vi "keyboard.NoteOn.vi"(8 "error in (no error)":errorcluster, 10 "Note":T1, 11 "midi-ui in":refnum<class "midi-ui.lvclass">) -> (0 "error out":errorcluster, 3 "midi-ui out":refnum<class "midi-ui.lvclass">)   [LabVIEW 2020, in "midi-ui.lvclass"]
uses:
  midi-ui.lvclass
  shared/midi note number.ctl
  midi-ui.lvclass/midi-ui.ctl
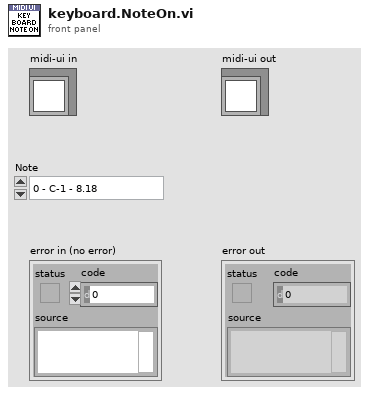
[diagram p1: front panel]
types:
  T1 = typedef "midi note number.ctl" = enum8{"0 - C-1 - 8.18", "1 - C#-1 - 8.66", "2 - D-1 - 9.18", "3 - D#-1 - 9.72", "4 - E-1 - 10.30", "5 - F-1 - 10.91", "6 - F#-1 - 11.56", "7 - G-1 - 12.25", "8 - G#-1 - 12.98", "9 - A-1 - 13.75", "10 - A#-1 - 14.57", "11 - B-1 - 15.43", "12 - C0 - 16.35", "13 - C#0 - 17.32", "14 - D0 - 18.35", "15 - D#0 - 19.45", "16 - E0 - 20.60", "17 - F0 - 21.83", "18 - F#0 - 23.12", "19 - G0 - 24.50", "20 - G#0 - 25.96", "21 - A0 - 27.50", "22 - A#0 - 29.14", "23 - B0 - 30.87", "24 - C1 - 32.70", "25 - C#1 - 34.65", "26 - D1 - 36.71", "27 - D#1 - 38.89", "28 - E1 - 41.20", "29 - F1 - 43.65", "30 - F#1 - 46.25", "31 - G1 - 49.00", "32 - G#1 - 51.91", "33 - A1 - 55.00", "34 - A#1 - 58.27", "35 - B1 - 61.74", "36 - C2 - 65.41", "37 - C#2 - 69.30", "38 - D2 - 73.42", "39 - D#2 - 77.78", "40 - E2 - 82.41", "41 - F2 - 87.31", "42 - F#2 - 92.50", "43 - G2 - 98.00", "44 - G#2 - 103.83", "45 - A2 - 110.00", "46 - A#2 - 116.54", "47 - B2 - 123.47", "48 - C3 - 130.81", "49 - C#3 - 138.59", "50 - D3 - 146.83", "51 - D#3 - 155.56", "52 - E3 - 164.81", "53 - F3 - 174.61", "54 - F#3 - 185.00", "55 - G3 - 196.00", "56 - G#3 - 207.65", "57 - A3 - 220.00", "58 - A#3 - 233.08", "59 - B3 - 246.94", "60 - C4 - 261.63", "61 - C#4 - 277.18", "62 - D4 - 293.66", "63 - D#4 - 311.13", "64 - E4 - 329.63", "65 - F4 - 349.23", "66 - F#4 - 369.99", "67 - G4 - 392.00", "68 - G#4 - 415.30", "69 - A4 - 440.00", "70 - A#4 - 466.16", "71 - B4 - 493.88", "72 - C5 - 523.25", "73 - C#5 - 554.37", "74 - D5 - 587.33", "75 - D#5 - 622.25", "76 - E5 - 659.25", "77 - F5 - 698.46", "78 - F#5 - 739.99", "79 - G5 - 783.99", "80 - G#5 - 830.61", "81 - A5 - 880.00", "82 - A#5 - 932.33", "83 - B5 - 987.77", "84 - C6 - 1046.50", "85 - C#6 - 1108.73", "86 - D6 - 1174.66", "87 - D#6 - 1244.51", "88 - E6 - 1318.51", "89 - F6 - 1396.91", "90 - F#6 - 1479.98", "91 - G6 - 1567.98", "92 - G#6 - 1661.22", "93 - A6 - 1760.00", "94 - A#6 - 1864.66", "95 - B6 - 1975.53", "96 - C7 - 2093.00", "97 - C#7 - 2217.46", "98 - D7 - 2349.32", "99 - D#7 - 2489.02", "100 - E7 - 2637.02", "101 - F7 - 2793.83", "102 - F#7 - 2959.96", "103 - G7 - 3135.96", "104 - G#7 - 3322.44", "105 - A7 - 3520.00", "106 - A#7 - 3729.31", "107 - B7 - 3951.07", "108 - C8 - 4186.01", "109 - C#8 - 4434.92", "110 - D8 - 4698.63", "111 - D#8 - 4978.03", "112 - E8 - 5274.04", "113 - F8 - 5587.65", "114 - F#8 - 5919.91", "115 - G8 - 6271.93", "116 - G#8 - 6644.88", "117 - A8 - 7040.00", "118 - A#8 - 7458.62", "119 - B8 - 7902.13", "120 - C9 - 8372.02", "121 - C#9 - 8869.84", "122 - D9 - 9397.27", "123 - D#9 - 9956.06", "124 - E9 - 10548.08", "125 - F9 - 11175.30", "126 - F#9 - 11839.82", "127 - G9 - 12543.85"}
  T2 = typedef "midi-ui.lvclass/privatedata.ctl" = cluster{"White Key Length":dbl, "White Key Width":dbl, "Black Key Length":dbl, "Key Polygon Corners by Name":map{string, cluster{"x":dbl, "y":dbl}[]}, "Anticlockwise rotations [0-3] (0)":i32, "Polygon Corners by Note Name":map{T1, cluster{"x":dbl, "y":dbl}[]}, "Picture Control":refnum<vi>, "Owning VI":refnum<vi>, "Control Index":i32, "Keyboard Key Note Bounds by Note Name":map{T1, cluster{"max":dbl, "min":dbl}}, "Notes on screen":cluster{"Note":T1, "End Time":u32, "Start Time":u32}[], "Polygon Pictures by Note Name":map{T1, cluster{"Note On":picture, "Note Off":picture}}, "keyboard":picture[], "Keyboard Note Picture Index by Name":map{T1, i32}, "music":picture[], "Zoom Factor":sgl, "keyboard - all off":picture[]}
  T3 = map{T1, cluster{"Note On":picture, "Note Off":picture}}
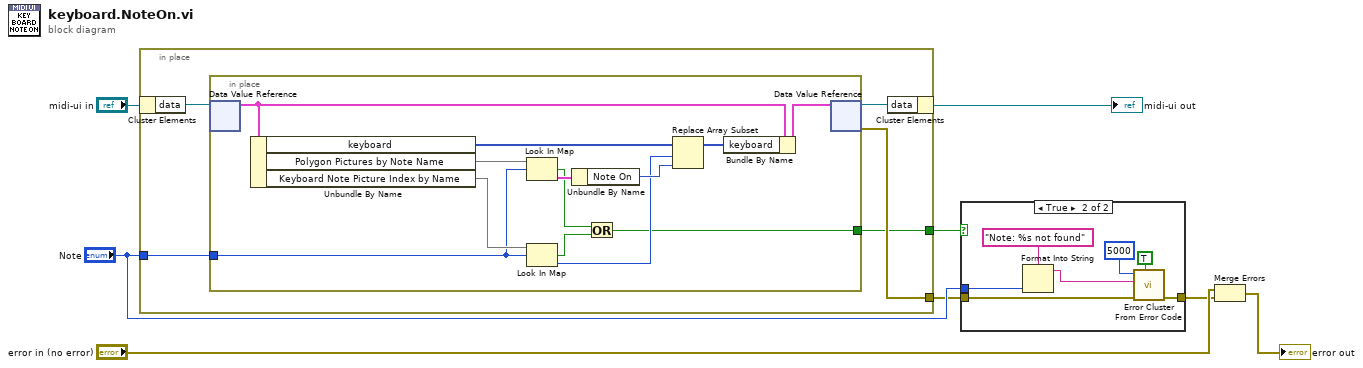
[diagram p0: block diagram]
diagram:
  n1 = in-place {
    in-place-border: "Note" -> [w13]
    in-place-border: [w10] -> w2
    in-place-border: [w9] -> w4
    n2 = in-place-cluster #1("midi-ui in") -> ("data"=w12:refnum<data-value>)
    n3 = in-place {
      in-place-border: w13 -> [w17]
      in-place-border: [w14] -> w9
      n4 = in-place-dvr #2(w12) -> (w20:T2)  [unwired: 1 out]
      n5 = Unbundle By Name(w20) -> ("keyboard"=w26:picture[], "Polygon Pictures by Note Name"=w22:T3, "Keyboard Note Picture Index by Name"=w21:map{T1, i32})
      n6 = Look In Map(map=w22, key=w17) -> (key not found?=w15:bool, value=w25:cluster{"Note On":picture, "Note Off":picture})  [unwired: 1 in]
      n7 = Look In Map(map=w21, key=w17) -> (key not found?=w16:bool, value=w23:i32)  [unwired: 1 in]
      n8 = Unbundle By Name(w25) -> ("Note On"=w24:picture)
      n9 = Or(x=w15, y=w16) -> (x .or. y?=w14:bool)
      n10 = Replace Array Subset(array=w26, new element=w24, index=w23) -> (w19:picture[])
      n11 = Bundle By Name(cluster=w20, "keyboard"=w19) -> (w18:T2)
      n12 = in-place-dvr #2(w18) -> (w11:refnum<data-value>, w10:errorcluster)
    }
    n13 = in-place-cluster #1("data"=w11) -> (→"midi-ui out":refnum<class "midi-ui.lvclass">)
  }
  n14 = case shown="True" w4 {
    tunnel: [w27 w34] -> w1
    tunnel: w2 -> [w27 w32]
    tunnel: "Note" -> [_ w29]
    frame False {
    }
    frame True {
      n15 = Format Into String(format string="Note: %s not found", w29) -> (resulting string=w28:string)  [unwired: 2 in, 1 out]
      n16 = call <vilib>:"Error Cluster From Error Code.vi"("show call chain? (False)"=TRUE, "error in (no error)"=w32, "error message (\"\")"=w28, "error code (0)"=5000) -> ("error out"=w34:errorcluster)  [unwired: 5 in]
    }
  }
  n17 = Merge Errors("error in (no error)", w1) -> (→"error out":errorcluster)
